vi "SDSU_DACS_Replace_Constant.vi"(5 "Field in":string, 7 "DAC name":string, 8 "error in (no error)":errorcluster, 9 "value  in":string, 10 "constants from file":string[][](table)) -> (0 "error out":errorcluster, 1 "value out":string, 2 "rest out":string)   [LabVIEW 2016]
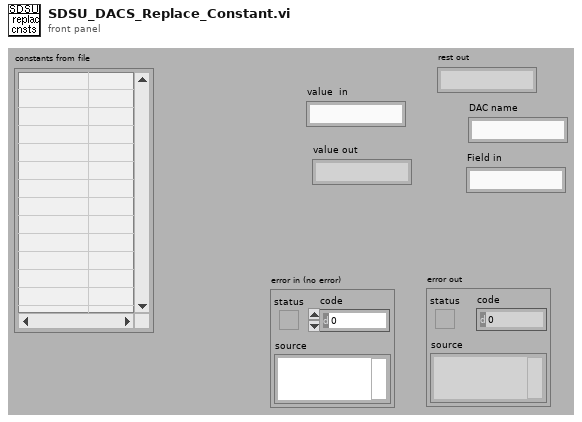
[diagram p1: front panel]
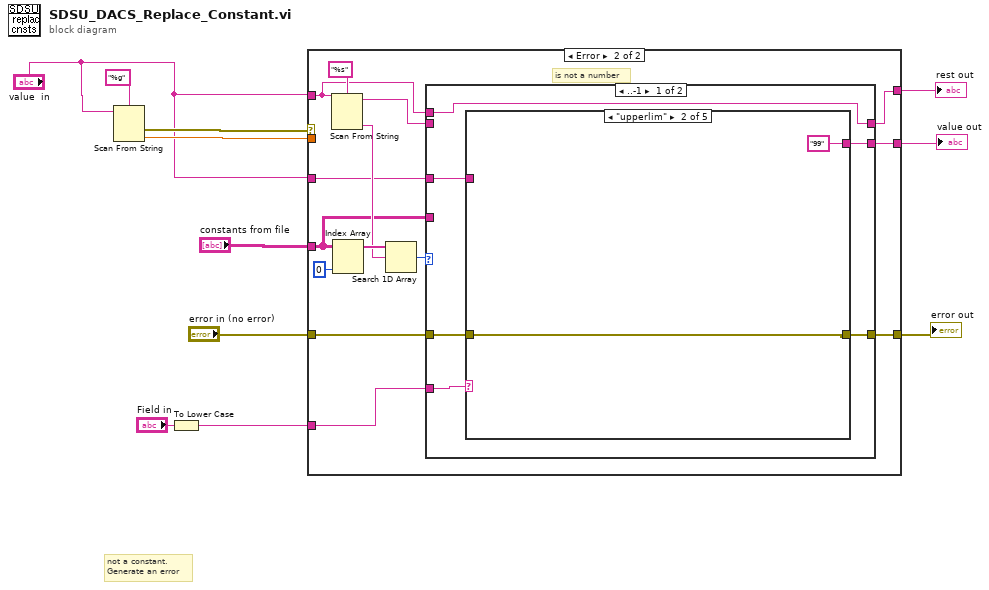
[diagram p0: block diagram]
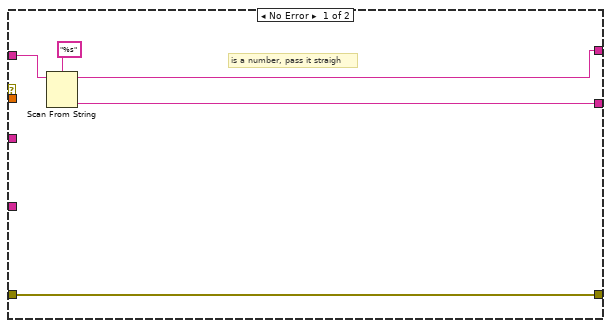
[diagram p2: hidden frame]
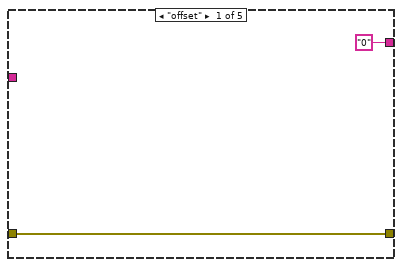
[diagram p3: hidden frame]
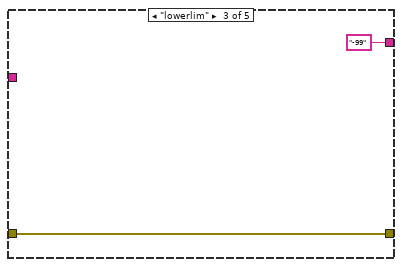
[diagram p4: hidden frame]
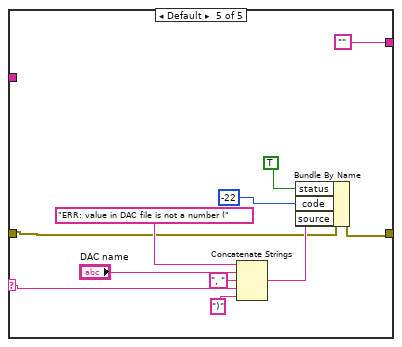
[diagram p6: hidden frame]
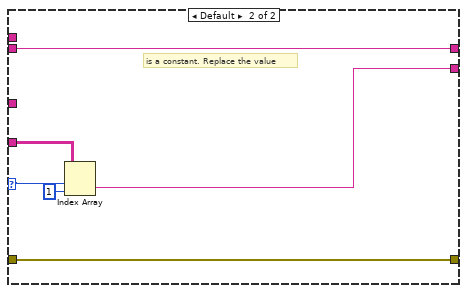
[diagram p7: hidden frame]
diagram:
  # "not a constant.\nGenerate an error"
  n1 = Scan From String(format string="%g", input string="value  in") -> (error out=w5:errorcluster, output 1=w4:dbl)  [unwired: 2 in, 3 out]
  n2 = To Lower Case(string="Field in") -> (all lower case string=w1:string)
  n3 = case shown="Error" w5 {
    tunnel: w4 -> [_ _]
    tunnel: "value  in" -> [w16 w17]
    tunnel: [w14 w22] -> w11
    tunnel: "error in (no error)" -> [w13 w25]
    tunnel: [w13 w24] -> w9
    tunnel: "constants from file" -> [_ w23]
    tunnel: w1 -> [_ w21]
    tunnel: "value  in" -> [_ w20]
    tunnel: [w12 w18] -> w6
    frame No Error {
      # "is a number, pass it straigh"
      n4 = Scan From String(format string="%s", input string=w16) -> (remaining string=w12:string, output 1=w14:string)  [unwired: 2 in, 3 out]
    }
    frame Error {
      # "is not a number"
      n5 = Scan From String(format string="%s", input string=w17) -> (remaining string=w19:string, output 1=w27:string)  [unwired: 2 in, 3 out]
      n6 = Index Array(array=w23, index (col)=0 ("disabled index (col)")) -> (element=w28:string[])  [unwired: 1 in]
      n7 = Search 1D Array(1D array=w28, element=w27) -> (index of element=w26:i32)  [unwired: 1 out]
      n8 = case shown="..-1" w26 {
        selector: w26 -> [_ w59]
        tunnel: w25 -> [w32 w61]
        tunnel: [w31 w61] -> w24
        tunnel: w23 -> [_ w60]
        tunnel: [w36 w57] -> w22
        tunnel: w21 -> [w34 _]
        tunnel: w20 -> [w35 _]
        tunnel: w19 -> [_ w56]
        tunnel: [w33 w56] -> w18
        tunnel: w17 -> [w33 _]
        frame ..-1 {
          n9 = case shown="\"upperlim\"" w34 {
            selector: w34 -> [_ _ _ _ w48]
            tunnel: ["0" "99" "-99" w44 ""] -> w36
            tunnel: w35 -> [_ _ _ w44 _]
            tunnel: w32 -> [w37 w39 w41 w43 w47]
            tunnel: [w37 w39 w41 w43 w46] -> w31
            frame "offset" {
            }
            frame "upperlim" {
            }
            frame "lowerlim" {
            }
            frame "comment" {
            }
            frame Default {
              n10 = Concatenate Strings("ERR: value in DAC file is not a number (" ("source"), "DAC name", ", " ("string"), w48, ")" ("string")) -> (w49:string)
              n11 = Bundle By Name(cluster=w47, "status"=TRUE, "code"=-22, "source"=w49) -> (w46:errorcluster)
            }
          }
        }
        frame Default {
          # "is a constant. Replace the value"
          n12 = Index Array(array=w60, index (row)=w59, index (col)=1 ("disabled index (col)")) -> (element=w57:string)
        }
      }
    }
  }
  "error out" <- w9
  "value out" <- w11
  "rest out" <- w6
